vi "Test_monitorCommand_setValue.vi"(8 "error in (no error)":errorcluster, 11 "command_setValue_Ctl":T1={"private_rcvStamp"=0.0, "parametersAndValues"="                                                                                                                                                                                                                                                                "}) -> (0 "error out":errorcluster, 2 "function return":i32, 3 "command_setValue_Ctl out":T1={"private_rcvStamp"=0.0, "parametersAndValues"="                                                                                                                                                                                                                                                                "})   [LabVIEW 2018, in "SALLV_Test.lvlib"]
doc: "int Test_shm_monitorCommand_setValueLV(Test_command_setValueLV *command_setValue_Ctl );"
uses:
  DataTypes/command_setValue.ctl
  SALLV_Test.lvlib
  SALLV_Test.so
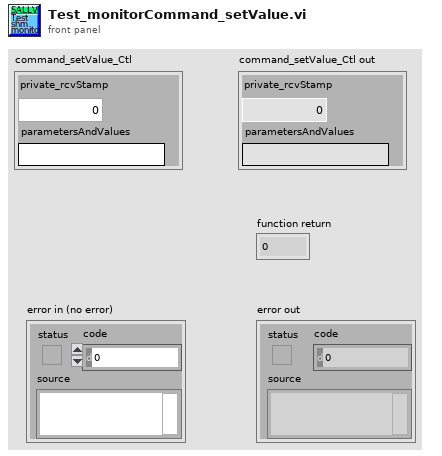
[diagram p1: front panel]
types:
  T1 = typedef "SALLV_Test.lvlib/command_setValue.ctl" = cluster{"private_rcvStamp":dbl, "parametersAndValues":string}
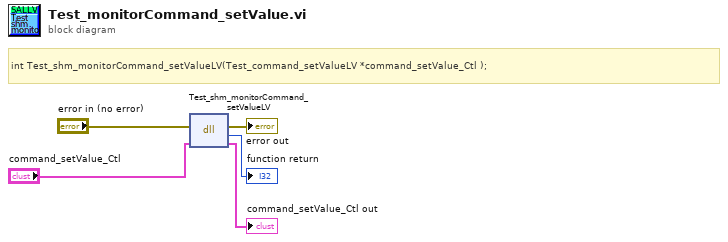
[diagram p0: block diagram]
diagram:
  # "int Test_shm_monitorCommand_setValueLV(Test_command_setValueLV *command_setValue_Ctl );"
  n1 = dll-call lib="home/ttsai/Documents/salTestLabViewApi/SALLV_Test/SALLV_Test.*" fn="Test_shm_monitorCommand_setValueLV"(error in="error in (no error)", "command_setValue_Ctl"="command_setValue_Ctl") -> (error out=→"error out":errorcluster, →"function return":i32, "command_setValue_Ctl"=→"command_setValue_Ctl out":T1)  [unwired: 2 in, 1 out]
